vi "Get Axis Motion Status Motor.vi"(8 "error in (no error)":errorcluster, 9 "Axis (1)":i32=1 min=1 max=3, 10 "VISA resource name":refnum<visa-resource-name>, 11 "ESP301 in":refnum<class "ESP301.lvclass">) -> (0 "error out":errorcluster, 1 "Motion Done":bool, 2 "VISA resource name out":refnum<visa-resource-name>, 3 "ESP301 out":refnum<class "ESP301.lvclass">)   [LabVIEW 2020, in "ESP301.lvclass"]
uses:
  ESP301.lvclass
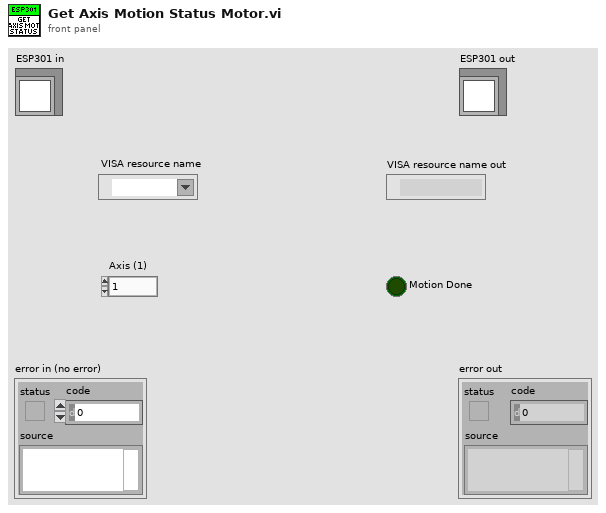
[diagram p1: front panel]
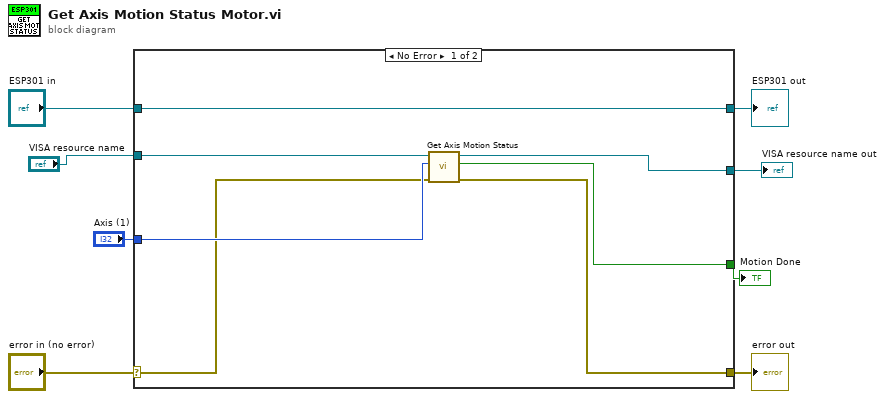
[diagram p0: block diagram]
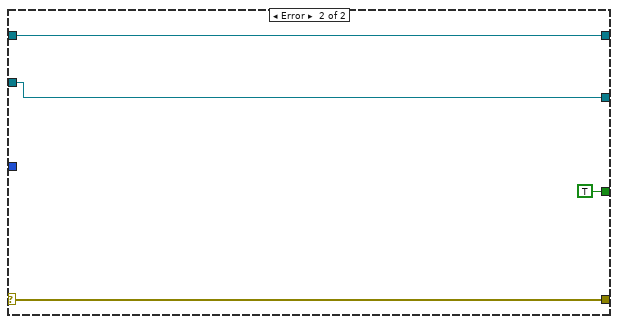
[diagram p2: hidden frame]
diagram:
  n1 = case shown="No Error" "error in (no error)" {
    selector: "error in (no error)" -> [w12 w19]
    tunnel: [w11 w19] -> w7
    tunnel: [w15 w18] -> w5
    tunnel: "ESP301 in" -> [w15 w18]
    tunnel: "VISA resource name" -> [w14 w17]
    tunnel: "Axis (1)" -> [w13 _]
    tunnel: [w10 w17] -> w2
    tunnel: [w9 TRUE ("Motion Done")] -> w1
    frame No Error {
      n2 = call "Get Axis Motion Status.vi"("error in (no error)"=w12, "Axis (1)"=w13, "VISA resource name"=w14) -> ("error out"=w11:errorcluster, "Motion Done"=w9:bool, "VISA resource name out"=w10:refnum<visa-resource-name>)  [unwired: 2 in]
    }
    frame Error {
    }
  }
  "error out" <- w7
  "ESP301 out" <- w5
  "VISA resource name out" <- w2
  "Motion Done" <- w1
